vi "get and set.vi"() -> ()   [LabVIEW 2013]
uses:
  errors/severity.ctl
  errors/const exceptioncausename.vi
  errors/const sourcename.vi
  errors/const messagename.vi
  errors/exception.lvlib
panel:
  out "call chain ok":bool
  out "src2 ok":bool
  out "msg2 ok":bool
  out "msg1 ok":bool
  out "src1 ok":bool
  out "cause ok":bool
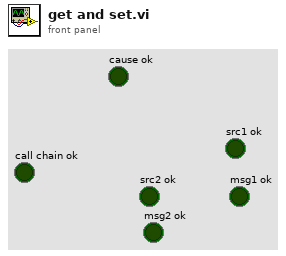
[diagram p1: front panel]
types:
  T1 = typedef "exception.lvlib/severity.ctl" = enum8{"unspecified", "operation failed", "data corruption", "system corruption", "critical unknown state"}
  T2 = typedef "exception.lvlib/exception.ctl" = cluster{"code":i32, "context":T3, "properties":variant}
  T3 = typedef "exception.lvlib/context.ctl" = enum16{"developer", "user interface", "standard", "limited", "deterministic"}
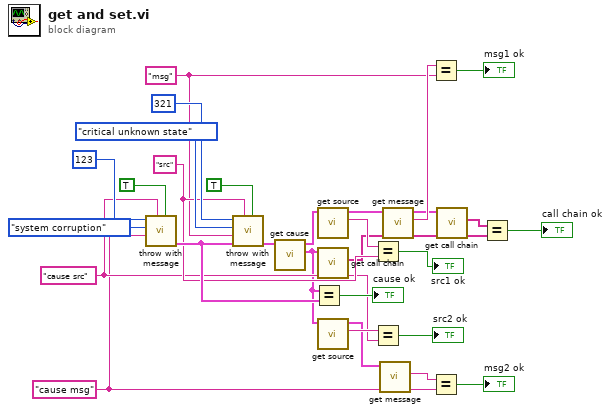
[diagram p0: block diagram]
diagram:
  w2 = "cause msg" ("message")
  w8 = "cause src" ("source")
  w1 = "msg" ("message")
  w16 = "src" ("source")
  n1 = call "throw with message.vi"("call chain?"=TRUE, "source"=w8, "message"=w2, "severity"=severity."system corruption", "code"=123) -> ("exception out"=w22:T2)  [unwired: 6 in]
  n2 = call "throw with message.vi"("call chain?"=TRUE, "source"=w16, "exception in"=w22, "message"=w1, "severity"=severity."critical unknown state", "code"=321) -> ("exception out"=w23:T2)  [unwired: 5 in]
  n3 = call "get cause.vi"("exception in"=w23) -> ("cause"=w6:T2, "exception out"=w20:T2)  [unwired: 9 in]
  n4 = Equal?(x=w6, y=w22) -> (x = y?=→"cause ok":bool)
  n5 = call "get source.vi"("exception in"=w20) -> ("source"=w17:string, "exception out"=w15:T2)  [unwired: 9 in]
  n6 = call "get call chain.vi"("exception in"=w6) -> ("call chain"=w4:string[])  [unwired: 9 in, 1 out]
  n7 = call "get source.vi"("exception in"=w6) -> ("source"=w12:string, "exception out"=w9:T2)  [unwired: 9 in]
  n8 = Equal?(x=w17, y=w16) -> (x = y?=→"src1 ok":bool)
  n9 = Equal?(x=w12, y=w8) -> (x = y?=→"src2 ok":bool)
  n10 = call "get message.vi"("exception in"=w9) -> ("message"=w13:string)  [unwired: 9 in, 1 out]
  n11 = call "get message.vi"("exception in"=w15) -> ("message"=w14:string, "exception out"=w7:T2)  [unwired: 9 in]
  n12 = Equal?(x=w14, y=w1) -> (x = y?=→"msg1 ok":bool)
  n13 = Equal?(x=w13, y=w2) -> (x = y?=→"msg2 ok":bool)
  n14 = call "get call chain.vi"("exception in"=w7) -> ("call chain"=w3:string[])  [unwired: 9 in, 1 out]
  n15 = Equal?(x=w3, y=w4) -> (x = y?=→"call chain ok":bool)
